vi "Get Simple Trigger Settings.vi"(8 "error in (no error)":errorcluster, 10 "Edge Trigger Settings":T2, 11 "PicoScope 3000a in":refnum<class "PicoScope 3000a.lvclass">) -> (0 "error out":errorcluster, 2 "Simple Trigger Settings":T3, 3 "PicoScope 3000a out":refnum<class "PicoScope 3000a.lvclass">)   [LabVIEW 2018, in "PicoScope 3000a.lvlib" / "PicoScope 3000a.lvclass"]
uses:
  PicoScope 3000a.lvclass
  PPLs/Oscilloscope/Parent/Oscilloscope.lvlibp/Custom Controls/Analog Channels.ctl
  Custom Controls/Simple Trigger Slope Direction.ctl
  PPLs/Oscilloscope/Parent/Oscilloscope.lvlibp
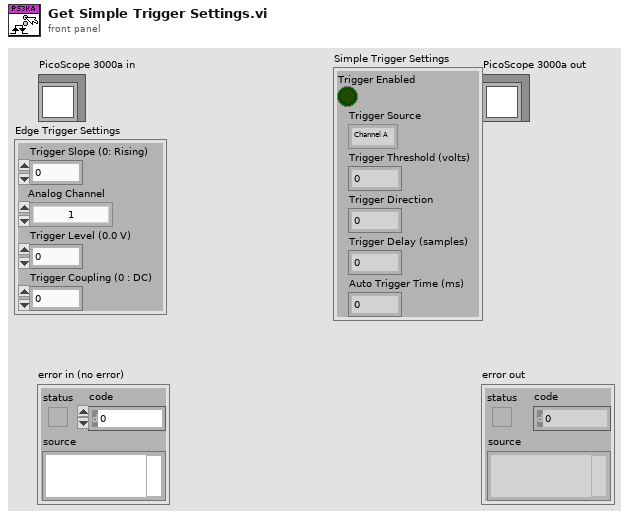
[diagram p1: front panel]
types:
  T1 = typedef "Oscilloscope.lvlibp/Analog Channels.ctl" = enum16{"1", "2", "3", "4", "5", "6", "7", "8", "9", "10", "11", "12", "13", "14", "15", "16"}
  T2 = cluster{"Trigger Slope (0: Rising)":u16, "Analog Channel":T1, "Trigger Level (0.0 V)":dbl, "Trigger Coupling (0 : DC)":u16}
  T3 = cluster{"Trigger Enabled":bool, "Trigger Source":enum32{"Channel A", "Channel B", "Channel C", "Channel D", "Ext."}, "Trigger Threshold (volts)":dbl, "Trigger Direction":u32, "Trigger Delay (samples)":u32, "Auto Trigger Time (ms)":i16}
  T4 = typedef "PicoScope 3000a.lvlib/PicoScope 3000a.lvclass/Simple Trigger Slope Direction.ctl" = enum16{"ABOVE", "BELOW", "RISING", "FALLING", "NEITHER"}
  T5 = enum32{"Channel A", "Channel B", "Channel C", "Channel D", "Ext."}
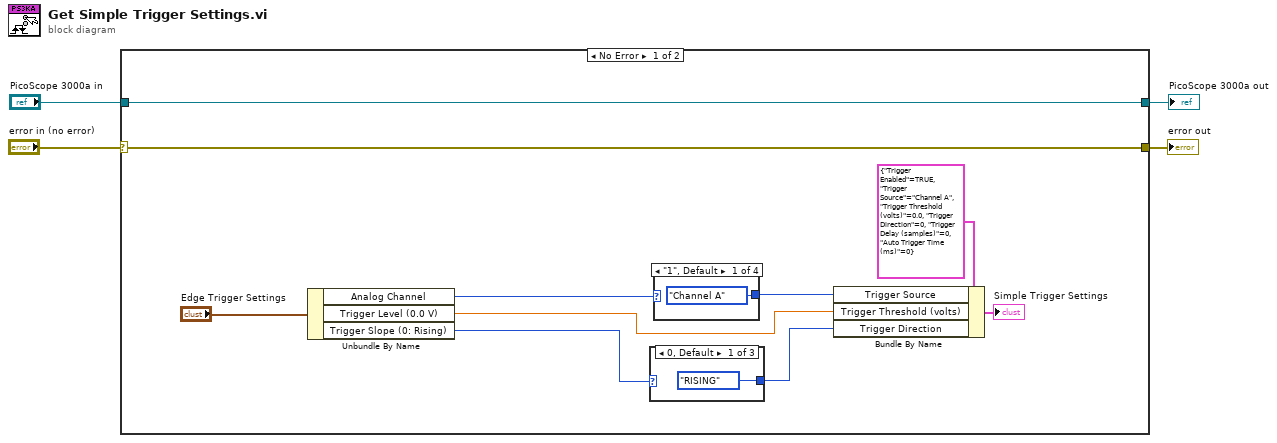
[diagram p0: block diagram]
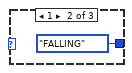
[diagram p2: hidden frame]
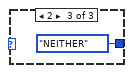
[diagram p3: hidden frame]
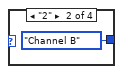
[diagram p4: hidden frame]
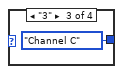
[diagram p5: hidden frame]
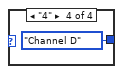
[diagram p6: hidden frame]
diagram:
  n1 = case shown="No Error" "error in (no error)" {
    selector: "error in (no error)" -> [w5 w23]
    tunnel: [w5 w23] -> w3
    tunnel: [w6 w22] -> w1
    tunnel: "PicoScope 3000a in" -> [w6 w22]
    frame No Error {
      n2 = Unbundle By Name("Edge Trigger Settings") -> ("Analog Channel"=w9:T1, "Trigger Level (0.0 V)"=w8:dbl, "Trigger Slope (0: Rising)"=w7:u16)
      n3 = case shown="0, Default" w7 {
        tunnel: [Simple_Trigger_Slope_Direction."RISING" ("Simple Trigger Slope Direction") Simple_Trigger_Slope_Direction."FALLING" ("Simple Trigger Slope Direction") Simple_Trigger_Slope_Direction."NEITHER" ("Simple Trigger Slope Direction")] -> w12
        frame 0, Default {
        }
        frame 1 {
        }
        frame 2 {
        }
      }
      n4 = case shown="\"1\", Default" w9 {
        tunnel: [T5."Channel A" ("Trigger Source") T5."Channel B" ("Trigger Source") T5."Channel C" ("Trigger Source") T5."Channel D" ("Trigger Source")] -> w13
        frame "1", Default {
        }
        frame "2" {
        }
        frame "3" {
        }
        frame "4" {
        }
      }
      n5 = Bundle By Name(cluster=T3 {"Trigger Enabled"=TRUE, "Trigger Source"=enum."Channel A", "Trigger Threshold (volts)"=0.0, "Trigger Direction"=0, "Trigger Delay (samples)"=0, "Auto Trigger Time (ms)"=0} ("Trigger Settings"), "Trigger Source"=w13, "Trigger Threshold (volts)"=w8, "Trigger Direction"=w12) -> (→"Simple Trigger Settings":T3)
    }
    frame Error {
    }
  }
  "error out" <- w3
  "PicoScope 3000a out" <- w1
